vi "Enumerate Chassis.vi"(6 "Map":map{string, T1}(c390), 8 "error in (no error)":errorcluster, 10 "Chassis Info":T1[](array[typedef]), 11 "Chassis Element":refnum<class "Config Element.lvclass">) -> (0 "error out":errorcluster, 2 "Chassis Element":refnum<class "Config Element.lvclass">[](array[class]))   [LabVIEW 2023, in "Volatus.lvlib" / "Hardware Info Module.lvclass"]
uses:
  Hardware Info Module.lvclass
  Hardware Info Module.lvclass/Hardware Info Module.ctl
  lv-cdm/CDM-Config/Config Element/Config Element.lvclass
  9117e1a3-44df-4d41-bfd4-07b4189bcc33.vi
  HW Info.ctl
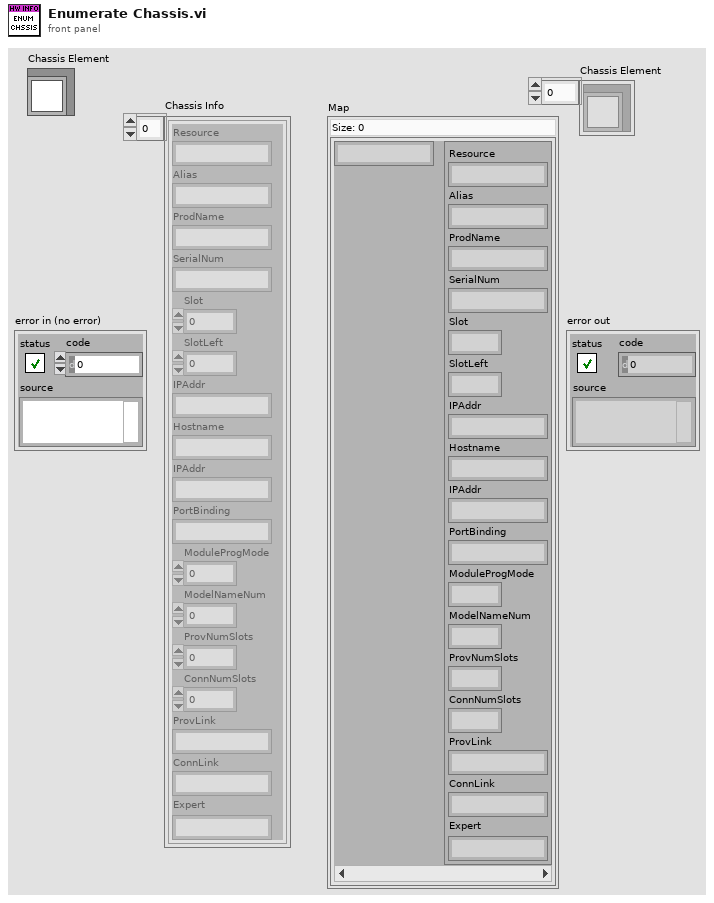
[diagram p1: front panel]
types:
  T1 = typedef "Volatus.lvlib/Hardware Info Module.lvclass/HW Info.ctl" = cluster{"Resource":string, "Alias":string, "ProdName":string, "SerialNum":string, "Slot":i32, "SlotLeft":u32, "IPAddr":string, "Hostname":string, "IPAddr":string, "PortBinding":string, "ModuleProgMode":u32, "ModelNameNum":u32, "ProvNumSlots":i32, "ConnNumSlots":i32, "ProvLink":string, "ConnLink":string, "Expert":string}
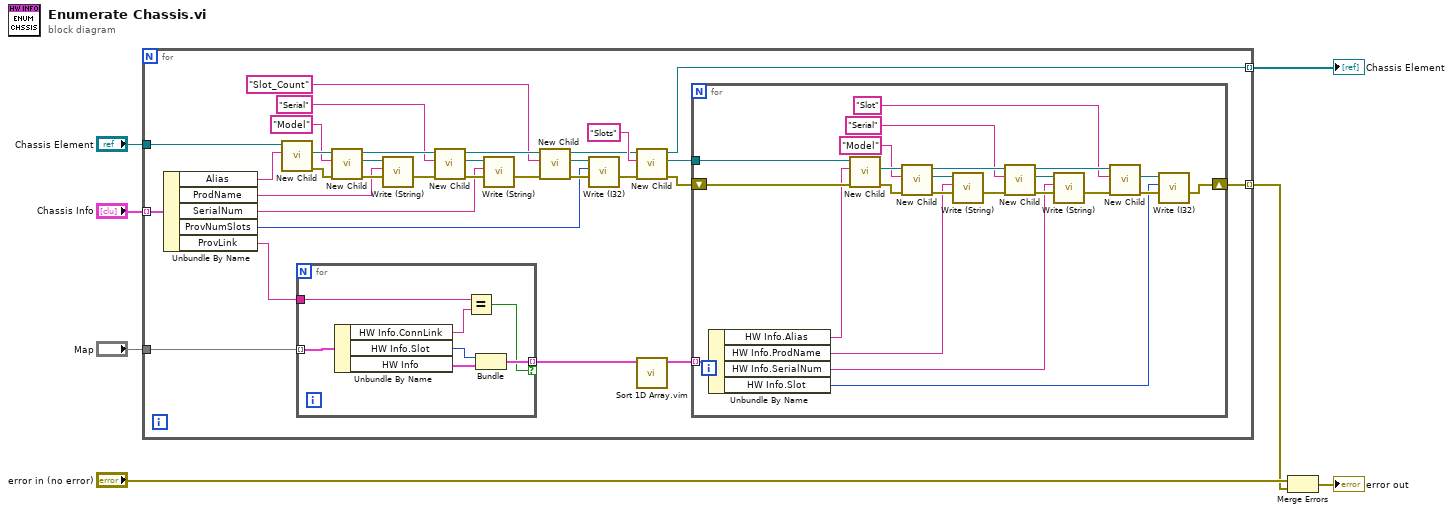
[diagram p0: block diagram]
diagram:
  n1 = for {
    tunnel: "Map" -> [w38]
    tunnel: "Chassis Element" -> [w37]
    tunnel: [w30] -> w3 mode=indexing
    tunnel: [w29] -> w2 mode=indexing
    tunnel: "Chassis Info" -> [w28] mode=indexing
    n2 = Unbundle By Name(w28) -> ("Alias"=w36:string, "ProdName"=w22:string, "SerialNum"=w16:string, "ProvNumSlots"=w10:i32, "ProvLink"=w39:string)
    n3 = call "New Child.vi"("Child Name"=w36, "Config Element in"=w37) -> ("error out"=w25:errorcluster, "New Child"=w27:refnum<class "Config Element.lvclass">)  [unwired: 7 in, 1 out]
    n4 = for {
      tunnel: w39 -> [w43]
      tunnel: w38 -> [w45] mode=indexing
      tunnel: [w42] -> w35 mode=indexing if=w41
      n5 = Unbundle By Name(w45) -> ("HW Info.ConnLink"=w44:string, "HW Info.Slot"=w46:i32, "HW Info"=w40:T1)
      n6 = Equal?(x=w43, y=w44) -> (x = y?=w41:bool)
      n7 = Bundle("Slot"=w46, "HW Info"=w40) -> (w42:cluster{"Slot":i32, "HW Info":T1})  [unwired: 1 in]
    }
    n8 = call "New Child.vi"("error in (no error)"=w25, "Child Name"="Model" ("Meta Name"), "Config Element in"=w27) -> ("error out"=w24:errorcluster, "New Child"=w23:refnum<class "Config Element.lvclass">, "Config Element out"=w18:refnum<class "Config Element.lvclass">)  [unwired: 6 in]
    n9 = call "Write (String).vi"("error in (no error)"=w24, "String Value"=w22, "Config Element in"=w23) -> ("error out"=w19:errorcluster)  [unwired: 7 in, 1 out]
    n10 = call "New Child.vi"("error in (no error)"=w19, "Child Name"="Serial" ("Meta Name"), "Config Element in"=w18) -> ("error out"=w20:errorcluster, "New Child"=w21:refnum<class "Config Element.lvclass">, "Config Element out"=w12:refnum<class "Config Element.lvclass">)  [unwired: 6 in]
    n11 = call "Write (String).vi"("error in (no error)"=w20, "String Value"=w16, "Config Element in"=w21) -> ("error out"=w13:errorcluster)  [unwired: 7 in, 1 out]
    n12 = call "New Child.vi"("error in (no error)"=w13, "Child Name"="Slot_Count" ("Meta Name"), "Config Element in"=w12) -> ("error out"=w15:errorcluster, "New Child"=w14:refnum<class "Config Element.lvclass">, "Config Element out"=w8:refnum<class "Config Element.lvclass">)  [unwired: 6 in]
    n13 = call "Write (I32).vi"("error in (no error)"=w15, "I32 Value"=w10, "Config Element in"=w14) -> ("error out"=w9:errorcluster)  [unwired: 7 in, 1 out]
    n14 = call "New Child.vi"("error in (no error)"=w9, "Child Name"="Slots" ("Meta Name"), "Config Element in"=w8) -> ("error out"=w31:errorcluster, "New Child"=w32:refnum<class "Config Element.lvclass">, "Config Element out"=w29:refnum<class "Config Element.lvclass">)  [unwired: 6 in]
    n15 = call "Sort 1D Array.vim"("unsorted array"=w35) -> ("sorted array"=w34:cluster{"Slot":i32, "HW Info":T1}[])  [unwired: 10 in]
    n16 = for {
      tunnel: w34 -> [w68] mode=indexing
      tunnel: w32 -> [w67]
      shift-right: [w47] -> w30
      shift-left: w31 -> [w69]
      n17 = Unbundle By Name(w68) -> ("HW Info.Alias"=w66:string, "HW Info.ProdName"=w52:string, "HW Info.SerialNum"=w50:string, "HW Info.Slot"=w48:i32)
      n18 = call "New Child.vi"("error in (no error)"=w69, "Child Name"=w66, "Config Element in"=w67) -> ("error out"=w54:errorcluster, "New Child"=w55:refnum<class "Config Element.lvclass">)  [unwired: 6 in, 1 out]
      n19 = call "New Child.vi"("error in (no error)"=w54, "Child Name"="Model" ("Meta Name"), "Config Element in"=w55) -> ("error out"=w56:errorcluster, "New Child"=w57:refnum<class "Config Element.lvclass">, "Config Element out"=w61:refnum<class "Config Element.lvclass">)  [unwired: 6 in]
      n20 = call "Write (String).vi"("error in (no error)"=w56, "String Value"=w52, "Config Element in"=w57) -> ("error out"=w60:errorcluster)  [unwired: 7 in, 1 out]
      n21 = call "New Child.vi"("error in (no error)"=w60, "Child Name"="Serial" ("Meta Name"), "Config Element in"=w61) -> ("error out"=w59:errorcluster, "New Child"=w58:refnum<class "Config Element.lvclass">, "Config Element out"=w65:refnum<class "Config Element.lvclass">)  [unwired: 6 in]
      n22 = call "Write (String).vi"("error in (no error)"=w59, "String Value"=w50, "Config Element in"=w58) -> ("error out"=w64:errorcluster)  [unwired: 7 in, 1 out]
      n23 = call "New Child.vi"("error in (no error)"=w64, "Child Name"="Slot" ("Meta Name"), "Config Element in"=w65) -> ("error out"=w62:errorcluster, "New Child"=w63:refnum<class "Config Element.lvclass">)  [unwired: 6 in, 1 out]
      n24 = call "Write (I32).vi"("error in (no error)"=w62, "I32 Value"=w48, "Config Element in"=w63) -> ("error out"=w47:errorcluster)  [unwired: 7 in, 1 out]
    }
  }
  "Chassis Element" <- w2
  n25 = Merge Errors("error in (no error)", w3) -> (→"error out":errorcluster)
